vi "Part Type to Fiducial Type.vi"(11 "Part Type":T2) -> (2 "Selection Strategy":T1, 3 "Fiducial Type":T3)   [LabVIEW 2011]
uses:
  Config Manager Class/Type Definitions/Fiducial Type.ctl
  Config Manager Class/Type Definitions/Part Type.ctl
  Config Manager Class/Type Definitions/Fiducial Selection Strategy.ctl
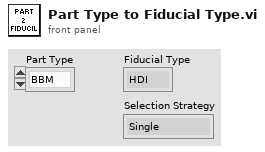
[diagram p1: front panel]
types:
  T1 = typedef "Fiducial Selection Strategy.ctl" = enum16{"Single", "Top", "Bottom"}
  T2 = typedef "Part Type.ctl" = enum16{"BBM", "HDI", "BARE HDI", "GLUERESERVOIR", "STAMP_1", "STAMP_2", "STAMP_3", "STAMP_4", "STAMP_5", "WEIGHT_1", "WEIGHT_2", "WEIGHT_3", "WEIGHT_4", "WEIGHT_5", "WEIGHT_6", "WEIGHT_7", "WEIGHT_8", "PICKER_TOOL", "GRABER_TOOL"}
  T3 = typedef "Fiducial Type.ctl" = enum16{"HDI", "BBM"}
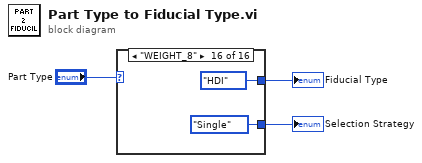
[diagram p0: block diagram]
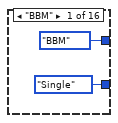
[diagram p2: hidden frame]
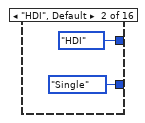
[diagram p3: hidden frame]
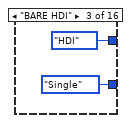
[diagram p4: hidden frame]
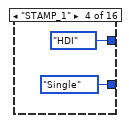
[diagram p5: hidden frame]
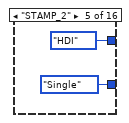
[diagram p6: hidden frame]
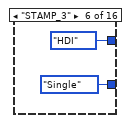
[diagram p7: hidden frame]
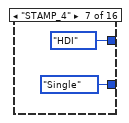
[diagram p8: hidden frame]
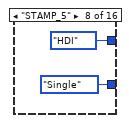
[diagram p9: hidden frame]
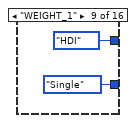
[diagram p10: hidden frame]
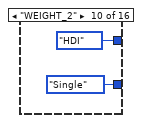
[diagram p11: hidden frame]
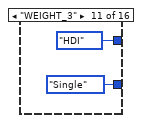
[diagram p12: hidden frame]
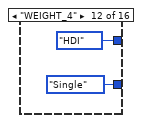
[diagram p13: hidden frame]
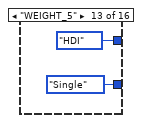
[diagram p14: hidden frame]
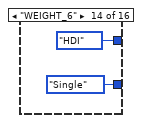
[diagram p15: hidden frame]
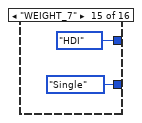
[diagram p16: hidden frame]
diagram:
  n1 = case shown="\"WEIGHT_8\"" "Part Type" {
    tunnel: [Fiducial_Type."BBM" ("Fiducial Type") Fiducial_Type."HDI" ("Fiducial Type") Fiducial_Type."HDI" ("Fiducial Type") Fiducial_Type."HDI" ("Fiducial Type") Fiducial_Type."HDI" ("Fiducial Type") Fiducial_Type."HDI" ("Fiducial Type") Fiducial_Type."HDI" ("Fiducial Type") Fiducial_Type."HDI" ("Fiducial Type") Fiducial_Type."HDI" ("Fiducial Type") Fiducial_Type."HDI" ("Fiducial Type") Fiducial_Type."HDI" ("Fiducial Type") Fiducial_Type."HDI" ("Fiducial Type") Fiducial_Type."HDI" ("Fiducial Type") Fiducial_Type."HDI" ("Fiducial Type") Fiducial_Type."HDI" ("Fiducial Type") Fiducial_Type."HDI" ("Fiducial Type")] -> w2
    tunnel: [Fiducial_Selection_Strategy."Single" ("Selection Criteria") Fiducial_Selection_Strategy."Single" ("Selection Criteria") Fiducial_Selection_Strategy."Single" ("Selection Criteria") Fiducial_Selection_Strategy."Single" ("Selection Criteria") Fiducial_Selection_Strategy."Single" ("Selection Criteria") Fiducial_Selection_Strategy."Single" ("Selection Criteria") Fiducial_Selection_Strategy."Single" ("Selection Criteria") Fiducial_Selection_Strategy."Single" ("Selection Criteria") Fiducial_Selection_Strategy."Single" ("Selection Criteria") Fiducial_Selection_Strategy."Single" ("Selection Criteria") Fiducial_Selection_Strategy."Single" ("Selection Criteria") Fiducial_Selection_Strategy."Single" ("Selection Criteria") Fiducial_Selection_Strategy."Single" ("Selection Criteria") Fiducial_Selection_Strategy."Single" ("Selection Criteria") Fiducial_Selection_Strategy."Single" ("Selection Criteria") Fiducial_Selection_Strategy."Single" ("Selection Criteria")] -> w1
    frame "BBM" {
    }
    frame "HDI", Default {
    }
    frame "BARE HDI" {
    }
    frame "STAMP_1" {
    }
    frame "STAMP_2" {
    }
    frame "STAMP_3" {
    }
    frame "STAMP_4" {
    }
    frame "STAMP_5" {
    }
    frame "WEIGHT_1" {
    }
    frame "WEIGHT_2" {
    }
    frame "WEIGHT_3" {
    }
    frame "WEIGHT_4" {
    }
    frame "WEIGHT_5" {
    }
    frame "WEIGHT_6" {
    }
    frame "WEIGHT_7" {
    }
    frame "WEIGHT_8" {
    }
  }
  "Fiducial Type" <- w2
  "Selection Strategy" <- w1
